vi "Check.vi"(8 "error in (no error)":errorcluster, 11 "Object License Manager in":refnum<class "Software License Manager.lvclass">) -> (0 "error out":errorcluster, 1 "ok?":bool, 2 "Body":string, 3 "Object License Manager out":refnum<class "Software License Manager.lvclass">)   [LabVIEW 2025, in "Software License Manager.lvclass"]
uses:
  Software License Manager.lvclass
  Software License Manager.lvclass/Software License Manager.ctl
  Board/Board.lvclass/Board.ctl
  Board/Read Product ID.vi
  <vilib>/httpClient/POSTBuffer.vi
  <vilib>/httpClient/LabVIEWHTTPClient.lvlib
  Board/Board.lvclass
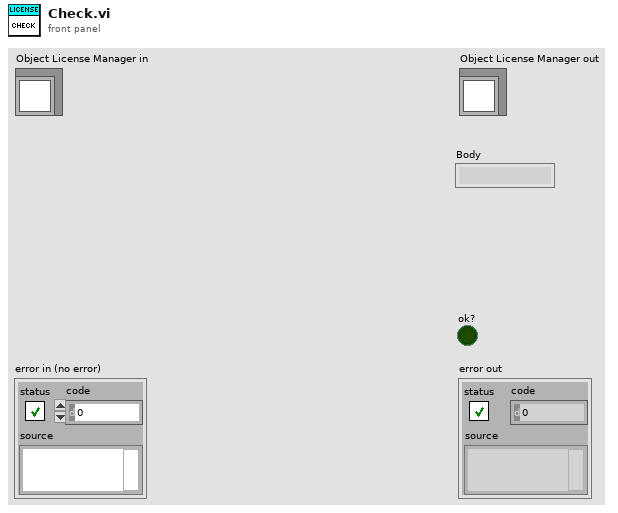
[diagram p1: front panel]
types:
  T1 = typedef "LabVIEWHTTPClient.lvlib/ClientHandle.ctl" = refnum<k1>
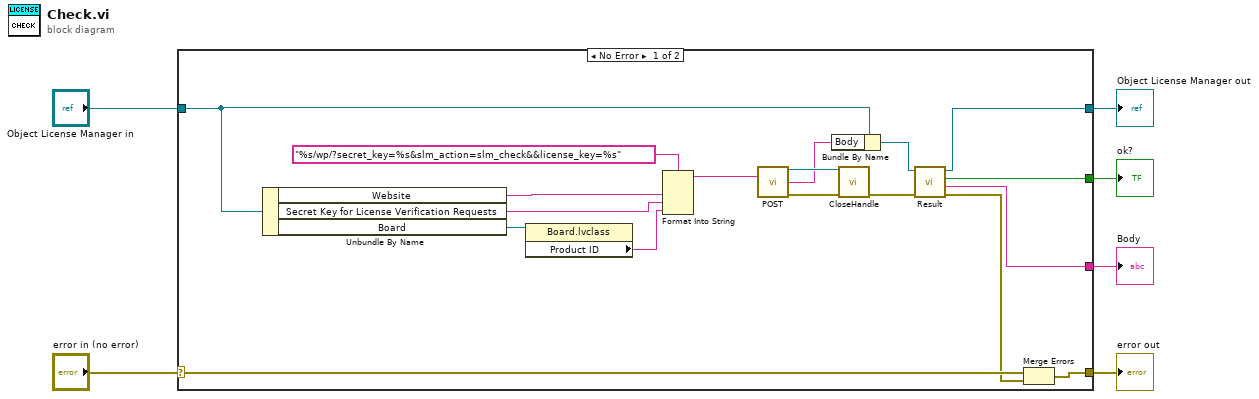
[diagram p0: block diagram]
diagram:
  n1 = case shown="No Error" "error in (no error)" {
    selector: "error in (no error)" -> [w24 w26]
    tunnel: [w10 w26] -> w5
    tunnel: [w12 w25] -> w3
    tunnel: "Object License Manager in" -> [w15 w25]
    tunnel: [w11 _] -> w2
    tunnel: [w8 _] -> w1
    frame No Error {
      n2 = Unbundle By Name(w15) -> ("Website"=w22:string, "Secret Key for License Verification Requests"=w7:string, "Board"=w21:refnum<class "Board.lvclass">)
      n3 = property class="Board.lvclass"(reference=w21) -> ("Product ID"=w20:string)  [unwired: 1 in, 2 out]
      n4 = Format Into String(format string="%s/wp/?secret_key=%s&slm_action=slm_check&&license_key=%s", w22, w7, w20) -> (resulting string=w19:string)  [unwired: 2 in, 1 out]
      n5 = call-poly <vilib>:"POST.vi"("url"=w19) -> ("client handle out"=w17:T1, "body"=w16:string, "error out"=w18:errorcluster)  [unwired: 11 in, 1 out]
      n6 = Bundle By Name(cluster=w15, "Body"=w16) -> (w13:refnum<class "Software License Manager.lvclass">)
      n7 = call <vilib>:"CloseHandle.vi"("client handle"=w17, "error in (no error)"=w18) -> ("error out"=w14:errorcluster)  [unwired: 13 in]
      n8 = call-dynamic "Result.vi"("error in (no error)"=w14, "Software License Manager in"=w13) -> ("error out"=w9:errorcluster, "Body"=w8:string, "ok?"=w11:bool, "Software License Manager out"=w12:refnum<class "Software License Manager.lvclass">)  [unwired: 6 in]
      n9 = Merge Errors(w24, w9) -> (w10:errorcluster)
    }
    frame Error {
    }
  }
  "error out" <- w5
  "Object License Manager out" <- w3
  "ok?" <- w2
  "Body" <- w1
